vi "Display Plugin UI in SubPanel.vi"(8 "error IO":errorcluster, 10 "VI reference":refnum<vi>, 11 "User Interface References":T1={"This VI"=refnum, "User Interace Plugin"=refnum, "UI Picture Container References"={"Header Image"=refnum, "Footer Image"=refnum}, "Sliding Menu XControl"=refnum, "Menu Container"=refnum, "UI Configuration Information"={"Space Between Buttons"=3, "Number of Buttons to Show"=6, "Header Image"=path "Images/Blue Background.bmp", "Footer Image"=path "Images/Blue Background.bmp"}, "Header Text"=refnum}) -> (0 "error out":errorcluster, 3 "User Interface References Out":T1={"This VI"=refnum, "User Interace Plugin"=refnum, "UI Picture Container References"={"Header Image"=refnum, "Footer Image"=refnum}, "Sliding Menu XControl"=refnum, "Menu Container"=refnum, "UI Configuration Information"={"Space Between Buttons"=3, "Number of Buttons to Show"=6, "Header Image"=path "Images/Blue Background.bmp", "Footer Image"=path "Images/Blue Background.bmp"}, "Header Text"=refnum})   [LabVIEW 2011, in "UI Load SubPanel Display.lvclass"]
uses:
  User Interface/UI Command Manager/UI Load SubPanel Display/UI Load SubPanel Display.lvclass
  Main Type Definitions/User Interface Type Definitions.ctl
  Main Type Definitions/UI Picture Containers.ctl
  Sliding Menu/Sliding Menu Library/Sliding Menu xControl/Sliding Menu XControl.xctl
  User Interface/UI Control Definitions/UI Configuration Information.ctl
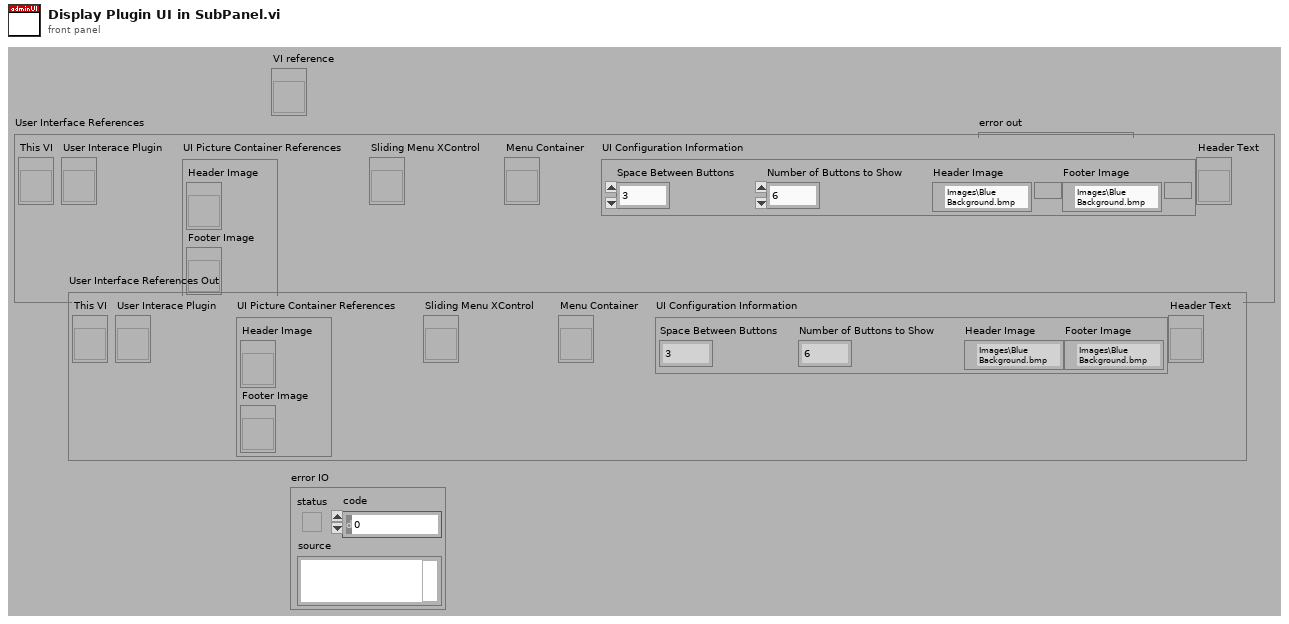
[diagram p1: front panel]
types:
  T1 = typedef "User Interface Type Definitions.ctl" = cluster{"This VI":refnum<vi>, "User Interace Plugin":refnum<vi>, "UI Picture Container References":T2, "Sliding Menu XControl":refnum<vi>, "Menu Container":refnum<vi>, "UI Configuration Information":T3, "Header Text":refnum<vi>}
  T2 = typedef "UI Picture Containers.ctl" = cluster{"Header Image":refnum<vi>, "Footer Image":refnum<vi>}
  T3 = typedef "UI Configuration Information.ctl" = cluster{"Space Between Buttons":i32, "Number of Buttons to Show":i32, "Header Image":path, "Footer Image":path}
  T4 = enum32{"invalid VI type", "Standard VI", "Control VI", "Global VI", "Polymorphic VI", "Configuration VI", "SubSystem", "Facade VI", "Method VI", "Statechart Diagram VI"}
  T5 = enum32{"Bad", "Idle", "Run top level", "Running"}
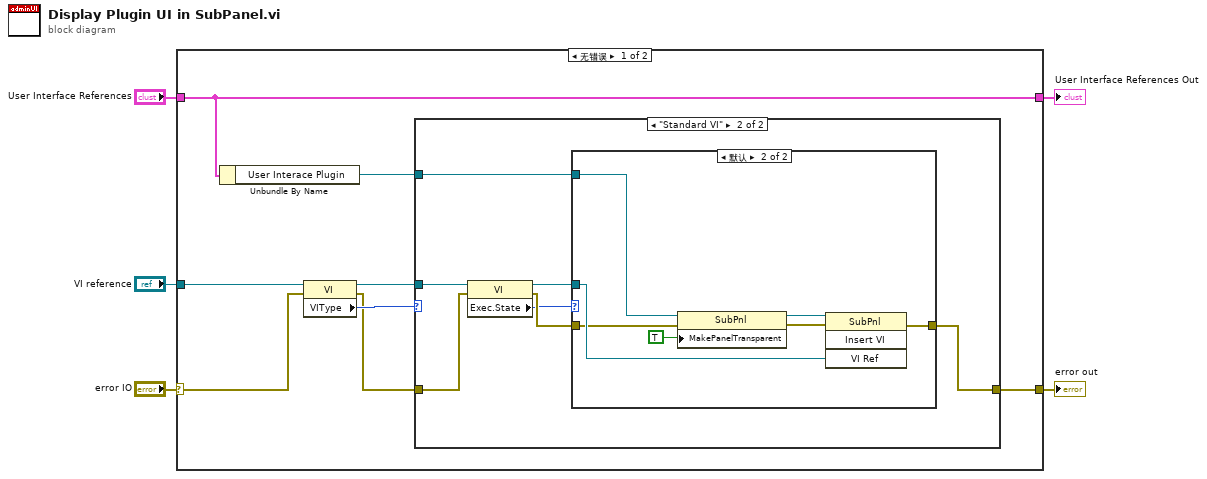
[diagram p0: block diagram]
diagram:
  n1 = case shown="无错误" "error IO" {
    selector: "error IO" -> [w9 w31]
    tunnel: [w10 w31] -> w5
    tunnel: "User Interface References" -> [w7 w30]
    tunnel: [w7 w30] -> w1
    tunnel: "VI reference" -> [w6 _]
    frame No Error {
      n2 = Unbundle By Name(w7) -> ("User Interace Plugin"=w11:refnum<vi>)
      n3 = property class="VI"(reference=w6, error in=w9) -> (reference out=w13:refnum<vi>, error out=w8:errorcluster, "VIType"=w12:T4)
      n4 = case shown="\"Standard VI\"" w12 {
        tunnel: [w14 w21] -> w10
        tunnel: w11 -> [_ w20]
        tunnel: w13 -> [_ w19]
        tunnel: w8 -> [w14 w18]
        frame "invalid VI type", Default {
        }
        frame "Standard VI" {
          n5 = property class="VI"(reference=w19, error in=w18) -> (reference out=w15:refnum<vi>, error out=w17:errorcluster, "Exec.State"=w16:T5)
          n6 = case shown="默认" w16 {
            tunnel: [w22 w26] -> w21
            tunnel: w20 -> [_ w25]
            tunnel: w15 -> [_ w24]
            tunnel: w17 -> [w22 w23]
            frame "Bad" {
            }
            frame Default {
              n7 = property class="SubPnl"(reference=w25, error in=w23, "MakePanelTransparent"=TRUE ("Panel Transparent")) -> (reference out=w28:refnum<vi>, error out=w29:errorcluster)
              n8 = invoke class="SubPnl" method="Insert VI"(reference=w28, error in=w29, "VI Ref"=w24) -> (error out=w26:errorcluster)  [unwired: 1 in, 3 out]
            }
          }
        }
      }
    }
    frame Error {
    }
  }
  "error out" <- w5
  "User Interface References Out" <- w1
